vi "Validate funct trig pulse width.vi"(9 "Requested trigger pulse width (ms)":dbl min=0.0 step=0.1, 11 "Trigger delay (sec)":dbl) -> (2 "functional acq. stimulus trigger pulse width (ms)":dbl format="%#_6f")   [LabVIEW 2020]
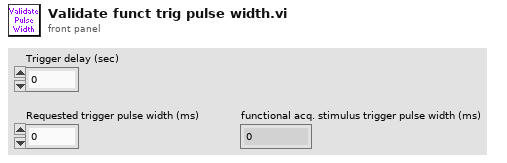
[diagram p1: front panel]
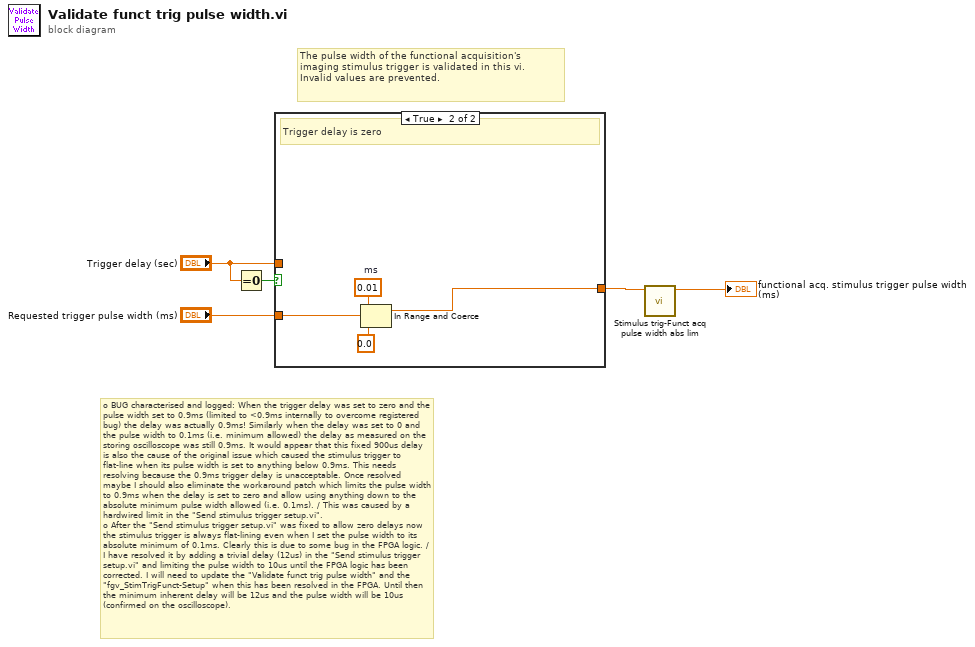
[diagram p0: block diagram]
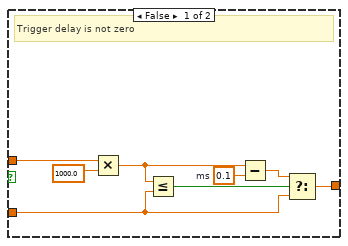
[diagram p2: hidden frame]
diagram:
  # "The pulse width of the functional acquisition's imaging stimulus trigger is validated in this vi.\nInvalid values are prevented."
  # "o\tBUG characterised and logged: When the trigger delay was set to zero and the pulse width set to 0.9ms (limited to <0.9ms internally to overcome registered bug) the delay was actually 0.9ms! Similarly when the delay was set to 0 and the pulse width to 0.1ms (i.e. minimum allowed) the delay as measured on the storing oscilloscope was still 0.9ms. It would appear that this fixed 900us delay is also the cause of the original issue which caused the stimulus trigger to flat-line when its pulse width is set to anything below 0.9ms. This needs resolving because the 0.9ms trigger delay is unacceptable. Once resolved maybe I should also eliminate the workaround patch which limits the pulse width to 0.9ms when the delay is set to zero and allow using anything down to the absolute minimum pulse width allowed (i.e. 0.1ms). / This was caused by a hardwired limit in the \"Send stimulus trigger setup.vi\".\no\tAfter the \"Send stimulus trigger setup.vi\" was fixed to allow zero delays now the stimulus trigger is always flat-lining even when I set the pulse width to its absolute minimum of 0.1ms. Clearly this is due to some bug in the FPGA logic. / I have resolved it by adding a trivial delay (12us) in the \"Send stimulus trigger setup.vi\" and limiting the pulse width to 10us until the FPGA logic has been corrected. I will need to update the \"Validate funct trig pulse width\" and the \"fgv_StimTrigFunct-Setup\" when this has been resolved in the FPGA. Until then the minimum inherent delay will be 12us and the pulse width will be 10us (confirmed on the oscilloscope)."
  n1 = Equal To 0?(x="Trigger delay (sec)") -> (x = 0?=w3:bool)
  n2 = case shown="True" w3 {
    tunnel: "Requested trigger pulse width (ms)" -> [w13 w15]
    tunnel: [w7 w14] -> w2
    tunnel: "Trigger delay (sec)" -> [w6 _]
    frame False {
      w8 = 0.1  # ms
      # "Trigger delay is not zero"
      n3 = Multiply(x=w6, y=1000.0) -> (x*y=w9:dbl)
      n4 = Less Or Equal?(x=w9, y=w13) -> (x <= y?=w11:bool)
      n5 = Subtract(x=w9, y=w8) -> (x-y=w12:dbl)
      n6 = Select(t=w12, s=w11, f=w13) -> (s? t:f=w7:dbl)
    }
    frame True {
      w17 = 0.01  # ms
      # "Trigger delay is zero"
      n7 = In Range and Coerce(upper limit=w17, x=w15, lower limit=0.0) -> (coerced(x)=w14:dbl)  [unwired: 1 out]
    }
  }
  n8 = call "Stimulus trig-Funct acq pulse width abs lim.vi"("Funct acq. stimulus trigger pulse width (ms)"=w2) -> ("Funct acq. stimulus trigger pulse width (ms)"=→"functional acq. stimulus trigger pulse width (ms)":dbl)  [unwired: 10 in]
